vi "FormatGraph.vi"(0 "Buffers in":T1={"Channels"=[], "PosttriggerBuffer"=refnum, "PretriggerBuffer"=refnum, "BlockSizePerChannel"=0, " logging semaphore"=refnum, "Log refnum"=refnum, "snapshotBuffer"=refnum, "logDirectory"=path "", "logPrefix"="", "decimation factor"=1, "max files"=0, "SampleRate"=0.0}, 1 "snapshotRef":refnum<vi>, 11 "error in (no error)":errorcluster) -> (4 "Buffers out":T1={"Channels"=[], "PosttriggerBuffer"=refnum, "PretriggerBuffer"=refnum, "BlockSizePerChannel"=0, " logging semaphore"=refnum, "Log refnum"=refnum, "snapshotBuffer"=refnum, "logDirectory"=path "", "logPrefix"="", "decimation factor"=1, "max files"=0, "SampleRate"=0.0}, 15 "error out":errorcluster)   [LabVIEW 2017]
uses:
  <vilib>/NI/PowerElectronicsControl/BufferLogging/Buffers.ctl
  <vilib>/NI/PowerElectronicsControl/BufferLogging/BufferLogging.lvlib
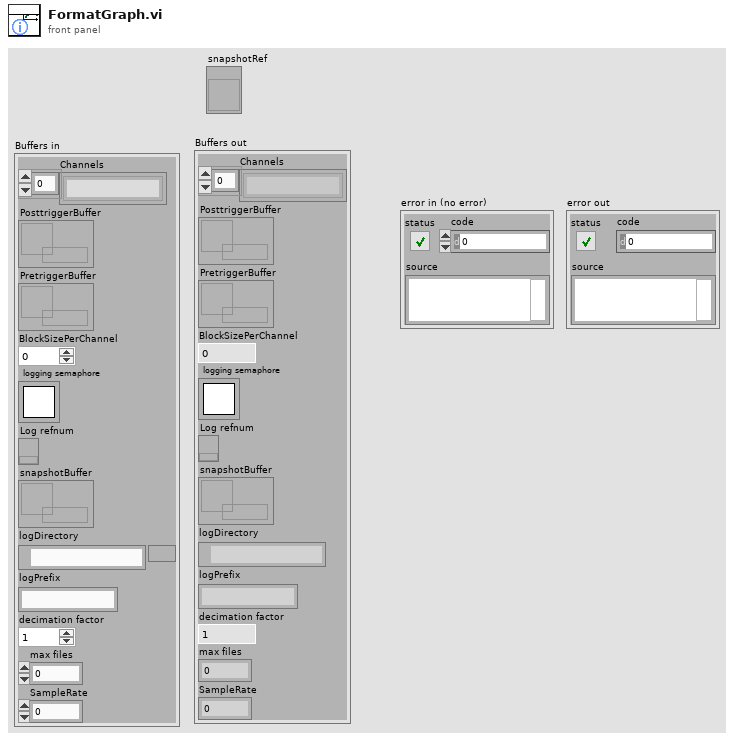
[diagram p1: front panel]
types:
  T1 = typedef "BufferLogging.lvlib/Buffers.ctl" = cluster{"Channels":string[], "PosttriggerBuffer":refnum<queue>, "PretriggerBuffer":refnum<queue>, "BlockSizePerChannel":i32, " logging semaphore":T2, "Log refnum":refnum<k34>, "snapshotBuffer":refnum<data-value>, "logDirectory":path, "logPrefix":string, "decimation factor":i32, "max files":i32, "SampleRate":dbl}
  T2 = typedef "Semaphore RefNum" = refnum<k1>
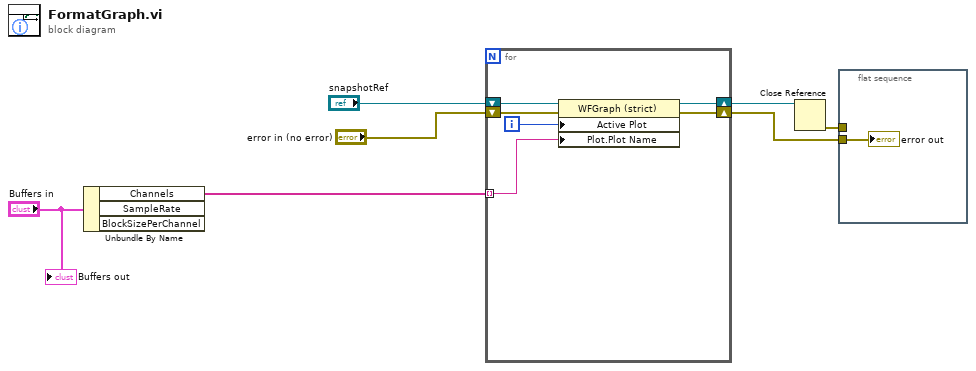
[diagram p0: block diagram]
diagram:
  n1 = Unbundle By Name("Buffers in") -> ("Channels"=w6:string[])  [unwired: 2 out]
  n2 = for {
    tunnel: w6 -> [w11] mode=indexing
    shift-right: [w10] -> w3
    shift-left: "snapshotRef" -> [w13]
    shift-right: [w8] -> w4
    shift-left: "error in (no error)" -> [w9]
    i -> [w12]
    n3 = property on="Property Node" class="WFGraph (strict)"(reference=w13, error in=w9, "Active Plot"=w12, "Plot.Plot Name"=w11) -> (reference out=w10:refnum<vi>, error out=w8:errorcluster)
  }
  n4 = Close Reference(reference=w3) -> (error out=w2:errorcluster)  [unwired: 1 in]
  n5 = flat-sequence {
    tunnel: w4 -> [w14]
    tunnel: w2 -> [_]
    frame #0 {
      "error out" <- w14
    }
  }
  "Buffers out" <- "Buffers in"
